vi "Wait for Client.vi"(8 "Error In":errorcluster, 11 "Listener Ref":refnum<k24>) -> (0 "Error Out":errorcluster, 3 "Client Ref":refnum<k24>)   [LabVIEW 2014, in "SSL Lib.lvlib"]
doc: "VI Function: This VI waits for a TCP client to connect to the TCP server.\n\nVI Version: 1.0\n\nVI Author: Runjhun Agarwal"
uses:
  <userlib>/SSL Library/SSL Lib.lvlib
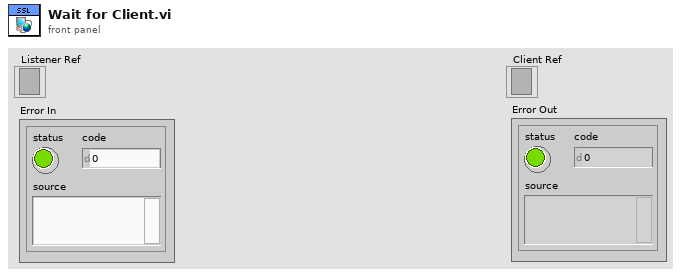
[diagram p1: front panel]
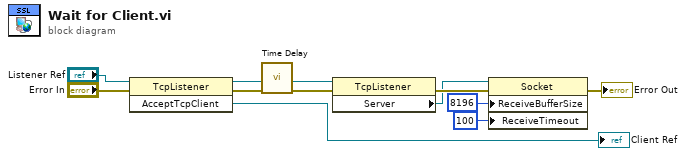
[diagram p0: block diagram]
diagram:
  n1 = invoke class="TcpListener" method="AcceptTcpClient"(reference="Listener Ref", error in="Error In") -> (reference out=w5:refnum<k24>, error out=w2:errorcluster, "AcceptTcpClient"=→"Client Ref":refnum<k24>)  [unwired: 1 in]
  n2 = call "Time Delay"("error in (no error)"=w2) -> ("error out"=w1:errorcluster)  [unwired: 10 in]
  n3 = property class="TcpListener"(reference=w5, error in=w1) -> (error out=w9:errorcluster, "Server"=w6:refnum<k24>)  [unwired: 1 out]
  n4 = property class="Socket"(reference=w6, error in=w9, "ReceiveBufferSize"=8196, "ReceiveTimeout"=100) -> (error out=→"Error Out":errorcluster)  [unwired: 1 out]
